vi "py_venv_init.vi"() -> (3 "Refnum out":refnum<k35>)   [LabVIEW 2023]
uses:
  <vilib>/Python/Open Venv Python Session.vi
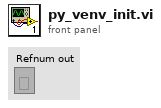
[diagram p1: front panel]
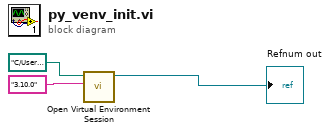
[diagram p0: block diagram]
diagram:
  n1 = call-poly <vilib>:"Open Virtual Environment Session.vi"("Python version"="3.10.0", "Env path"=path "C:/Users/bjohnst1/Documents/biomech_res/res_env2") -> ("session out"=→"Refnum out":refnum<k35>)  [unwired: 8 in, 1 out]
